vi "SuperSimpleEncoderTest.vi"() -> ()   [LabVIEW 2009]
uses:
  <vilib>/eio/EIONode/EIONode.xnode
  <vilib>/rvi/eio/nirviEIOImplementation/nirviEIOImplementation.xnode
  <vilib>/rvi/eio/common/nirviEmuTemplateMethod_noerrors.vi
  <vilib>/rvi/eio/common/nirviEmuClasses.ctl
panel:
  out "Steering Encoder A":bool
  out "Steering Encoder B":bool
  out "Steering Encoder Index":bool
  out "Lidar Encoder A":bool
  out "Lidar Encoder B":bool
  out "Lidar Encoder Index":bool
  out "Drive Encoder A":bool
  out "Drive Encoder B":bool
  out "Drive Encoder Index":bool
  in  "stop":bool
  in  "Lidar Enable":bool
  in  "Steering Enable":bool
  in  "Drive Enable":bool
  in  "Lidar output Voltage":fxp<+/-,20,5>
  in  "Steering output Voltage":fxp<+/-,20,5>
  in  "Drive output Voltage":fxp<+/-,20,5>
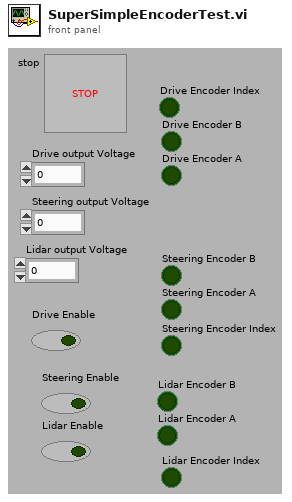
[diagram p1: front panel]
types:
  T1 = typedef "nirviEmuClasses.ctl" = enum16{"IO Read", "IO Write", "Method", "Property Read", "Property Write"}
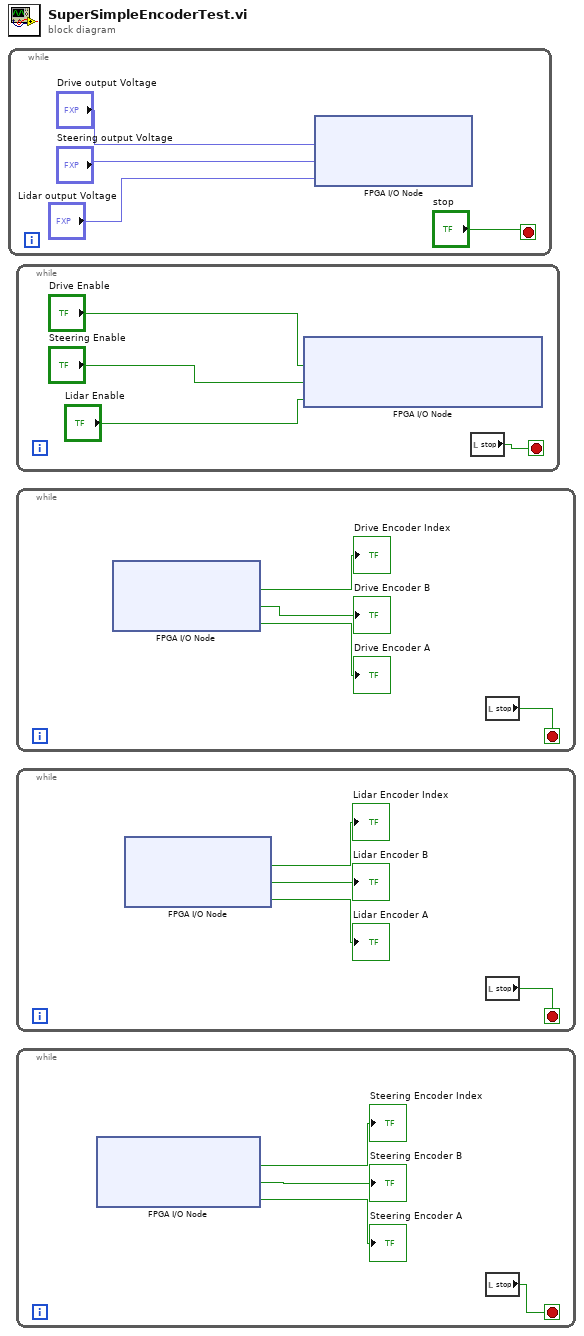
[diagram p0: block diagram]
diagram:
  n1 = while {
    stop <- "stop" stop-if-true
    n2 = xnode "FPGA I/O Node"("Drive Motor Speed"="Drive output Voltage", "Steering Motor Speed"="Steering output Voltage", "Lidar Motor Speed"="Lidar output Voltage") -> ()  [unwired: 3 in, 3 out]
  }
  n3 = while {
    stop <- w38 stop-if-true
    n4 = xnode "FPGA I/O Node"("Drive Motor Inhibit (Non-Functional)"="Drive Enable", "Steering Motor Inhibit"="Steering Enable", "Lidar Motor Inhibit"="Lidar Enable") -> ()  [unwired: 3 in, 3 out]
    n5 = local read "stop"() -> (w38:bool)
  }
  n6 = while {
    stop <- w78 stop-if-true
    n7 = xnode "FPGA I/O Node"() -> ("Drive Encoder Index"=→"Drive Encoder Index":bool, "Drive Encoder B"=→"Drive Encoder B":bool, "Steering Encoder A"=→"Drive Encoder A":bool)  [unwired: 3 in, 3 out]
    n8 = local read "stop"() -> (w78:bool)
  }
  n9 = while {
    stop <- w139 stop-if-true
    n10 = xnode "FPGA I/O Node"() -> ("Lidar Encoder Index"=→"Lidar Encoder Index":bool, "Lidar Encoder B"=→"Lidar Encoder B":bool, "Lidar Encoder A"=→"Lidar Encoder A":bool)  [unwired: 3 in, 3 out]
    n11 = local read "stop"() -> (w139:bool)
  }
  n12 = while {
    stop <- w200 stop-if-true
    n13 = xnode "FPGA I/O Node"() -> ("Steering Encoder Index"=→"Steering Encoder Index":bool, "Steering Encoder B"=→"Steering Encoder B":bool, "Port1/DIO9"=→"Steering Encoder A":bool)  [unwired: 3 in, 3 out]
    n14 = local read "stop"() -> (w200:bool)
  }
